vi "INTELLIFAUCET Driver.vi"(0 "VISA session":refnum<visa-resource-name>="MW100", 1 "Mode":T2=enum."Stop Flow", 2 "Use General Conversion":bool, 5 "Temperature(F)":dbl(slide)=58.0 scale=40.0..120.0, 7 "Flow Rate (GPM)":dbl(slide)=100.0 scale=0.0..100.0, 9 "uA Set":i32, 11 "Error In":errorcluster, 12 "Debug":bool, 13 "Refnum in":T1, 14 "Use Proportion Valve":bool) -> (4 "VISA session out":refnum<visa-resource-name>, 6 "Intellif Valve % Open":dbl, 8 "uA Output":i32, 15 "Error Out":errorcluster)   [LabVIEW 2016]
uses:
  Type Definitions/INTELLIFAUCET Set Mode.ctl
  Type Definitions/INTELLIFAUCT Temp Flow.ctl
panel:
  in  "milliseconds to wait":u32=25
  out "Local?":bool
  # "%"
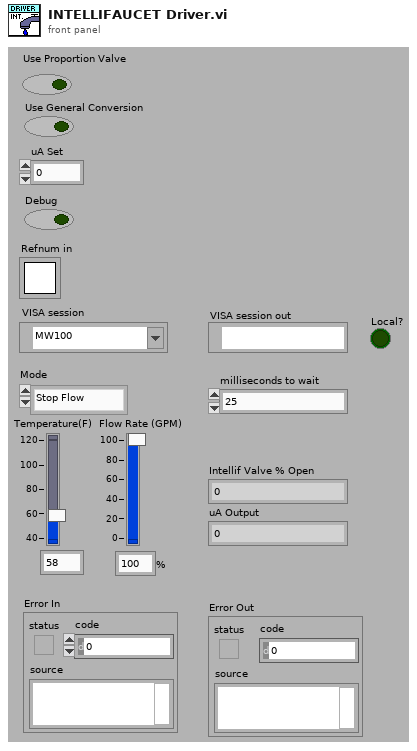
[diagram p1: front panel]
types:
  T1 = typedef "Semaphore RefNum" = refnum<k1>
  T2 = typedef "INTELLIFAUCET Set Mode.ctl" = enum16{"Adjust Temp", "Adjust Flow", "Start Flow", "Stop Flow", "Hold"}
  T3 = typedef "INTELLIFAUCT Temp Flow.ctl" = enum8{"TEMP", "FLOW"}
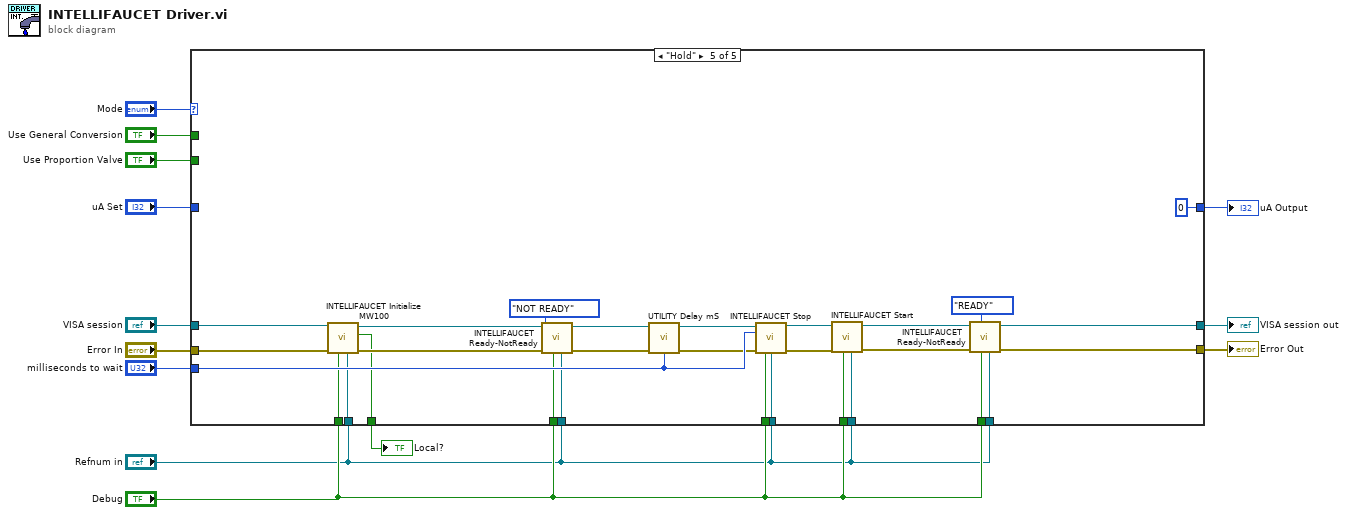
[diagram p0: block diagram]
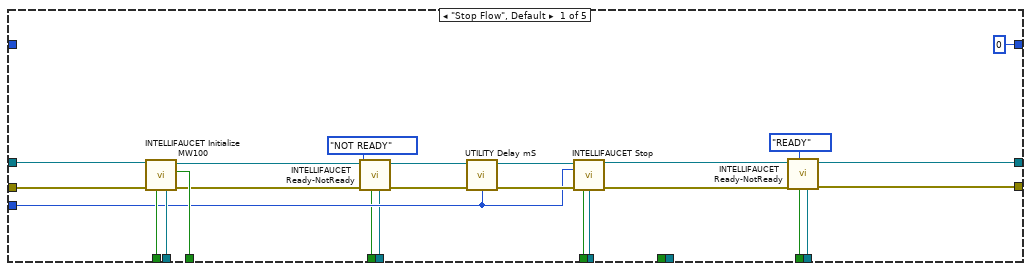
[diagram p2: hidden frame]
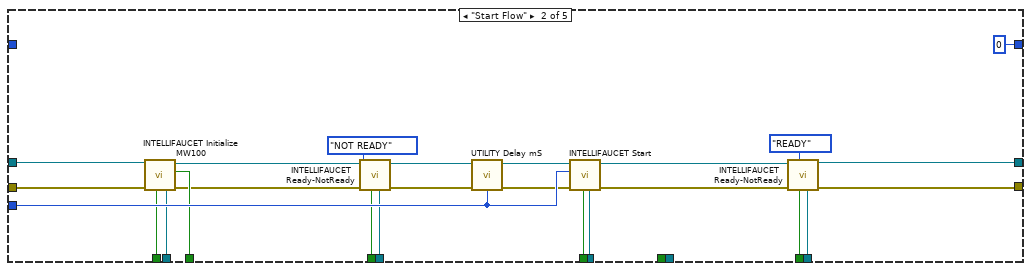
[diagram p3: hidden frame]
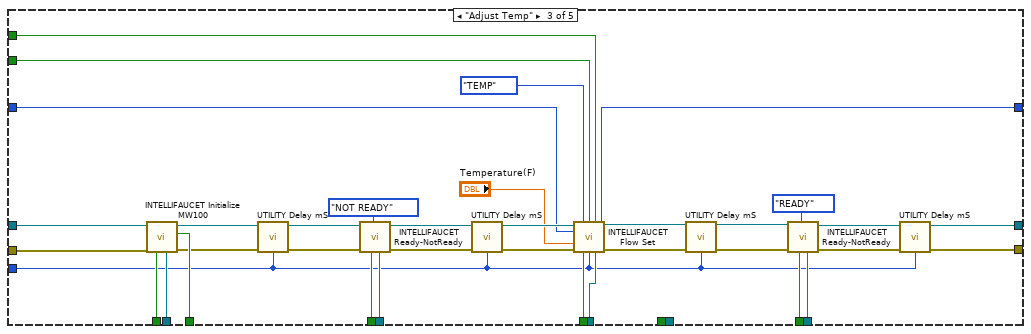
[diagram p4: hidden frame]
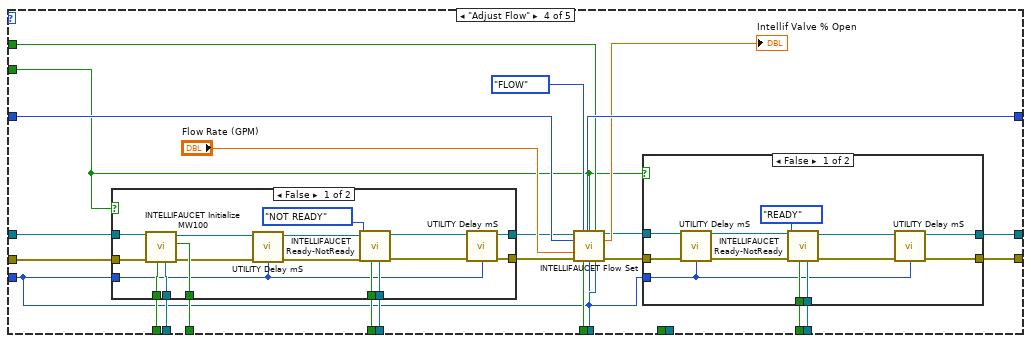
[diagram p5: hidden frame]
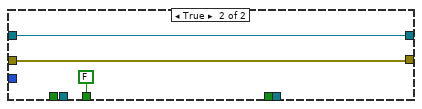
[diagram p7: hidden frame]
diagram:
  n1 = case shown="\"Hold\"" "Mode" {
    tunnel: "milliseconds to wait" -> [w28 w61 w65 w102 w168]
    tunnel: [w16 w46 w86 w115 w159] -> w10
    tunnel: "VISA session" -> [w35 w60 w84 w118 w170]
    tunnel: "Error In" -> [w36 w59 w85 w112 w169]
    tunnel: [w17 w45 w82 w117 w160] -> w11
    tunnel: [w34 w58 w81 w116 w163] -> w9
    tunnel: "Debug" -> [w26 w44 w78 w110 w165]
    tunnel: "Refnum in" -> [w25 w43 w77 w111 w164]
    tunnel: "Refnum in" -> [w32 w57 w79 w114 w166]
    tunnel: "Debug" -> [w33 w56 w80 w113 w167]
    tunnel: "Refnum in" -> [w30 w54 w75 w109 w161]
    tunnel: "Debug" -> [w31 w55 w76 w108 w162]
    tunnel: "Debug" -> [w15 w42 w74 w107 w158]
    tunnel: "Refnum in" -> [w14 w41 w73 w106 w157]
    tunnel: [0 ("uA Output") 0 ("uA Output") w72 w105 0 ("uA Output")] -> w8
    tunnel: "Use General Conversion" -> [_ _ w71 w103 _]
    tunnel: "uA Set" -> [_ _ w70 w104 _]
    tunnel: "Use Proportion Valve" -> [_ _ w62 w94 _]
    tunnel: "Debug" -> [_ _ _ _ w151]
    tunnel: "Refnum in" -> [_ _ _ _ w150]
    frame "Stop Flow", Default {
      n2 = call "INTELLIFAUCET Initialize MW100.vi"("Refnum in"=w32, "Debug"=w33, "error in (no error)"=w36, "MW100 Input"=w35) -> ("error out"=w24:errorcluster, "Local?"=w34:bool, "MW100 Output"=w22:refnum<visa-resource-name>)  [unwired: 5 in]
      n3 = call "INTELLIFAUCET Ready-NotReady.vi"("Refnum in"=w25, "Debug"=w26, "Error In"=w24, "READY?"=enum8{"READY", "NOT READY"}."NOT READY", "VISA session"=w22) -> ("Error Out"=w23:errorcluster, "dup VISA session"=w21:refnum<visa-resource-name>)  [unwired: 5 in]
      n4 = call "UTILITY Delay mS.vi"("Error In"=w23, "milliseconds to wait"=w28) -> ("Error Out"=w37:errorcluster)  [unwired: 13 in]
      n5 = call "INTELLIFAUCET Stop.vi"("VISA session"=w21, "mS wait"=w28, "Error In"=w37, "Debug"=w31, "Refnum in"=w30) -> ("dup VISA session"=w19:refnum<visa-resource-name>, "Error Out"=w18:errorcluster)  [unwired: 9 in]
      n6 = call "INTELLIFAUCET Ready-NotReady.vi"("Refnum in"=w14, "Debug"=w15, "Error In"=w18, "READY?"=enum8{"READY", "NOT READY"}."READY", "VISA session"=w19) -> ("Error Out"=w16:errorcluster, "dup VISA session"=w17:refnum<visa-resource-name>)  [unwired: 5 in]
    }
    frame "Start Flow" {
      n7 = call "INTELLIFAUCET Initialize MW100.vi"("Refnum in"=w57, "Debug"=w56, "error in (no error)"=w59, "MW100 Input"=w60) -> ("error out"=w38:errorcluster, "Local?"=w58:bool, "MW100 Output"=w51:refnum<visa-resource-name>)  [unwired: 5 in]
      n8 = call "INTELLIFAUCET Ready-NotReady.vi"("Refnum in"=w43, "Debug"=w44, "Error In"=w38, "READY?"=enum8{"READY", "NOT READY"}."NOT READY", "VISA session"=w51) -> ("Error Out"=w40:errorcluster, "dup VISA session"=w50:refnum<visa-resource-name>)  [unwired: 5 in]
      n9 = call "UTILITY Delay mS.vi"("Error In"=w40, "milliseconds to wait"=w61) -> ("Error Out"=w39:errorcluster)  [unwired: 13 in]
      n10 = call "INTELLIFAUCET Start.vi"("Refnum in"=w54, "Debug"=w55, "Error In"=w39, "mS wait"=w61, "VISA session"=w50) -> ("Error Out"=w47:errorcluster, "dup VISA session"=w48:refnum<visa-resource-name>)  [unwired: 5 in]
      n11 = call "INTELLIFAUCET Ready-NotReady.vi"("Refnum in"=w41, "Debug"=w42, "Error In"=w47, "READY?"=enum8{"READY", "NOT READY"}."READY", "VISA session"=w48) -> ("Error Out"=w46:errorcluster, "dup VISA session"=w45:refnum<visa-resource-name>)  [unwired: 5 in]
    }
    frame "Adjust Temp" {
      n12 = call "INTELLIFAUCET Initialize MW100.vi"("Refnum in"=w79, "Debug"=w80, "error in (no error)"=w85, "MW100 Input"=w84) -> ("error out"=w67:errorcluster, "Local?"=w81:bool, "MW100 Output"=w83:refnum<visa-resource-name>)  [unwired: 5 in]
      n13 = call "UTILITY Delay mS.vi"("Error In"=w67, "milliseconds to wait"=w65) -> ("Error Out"=w66:errorcluster)  [unwired: 13 in]
      n14 = call "INTELLIFAUCET Ready-NotReady.vi"("Refnum in"=w77, "Debug"=w78, "Error In"=w66, "READY?"=enum8{"READY", "NOT READY"}."NOT READY", "VISA session"=w83) -> ("Error Out"=w69:errorcluster, "dup VISA session"=w91:refnum<visa-resource-name>)  [unwired: 5 in]
      n15 = call "UTILITY Delay mS.vi"("Error In"=w69, "milliseconds to wait"=w65) -> ("Error Out"=w68:errorcluster)  [unwired: 13 in]
      n16 = call "INTELLIFAUCET Flow Set.vi"("VISA Refnum in"=w91, "TEMP,FLOW"=INTELLIFAUCT_Temp_Flow."TEMP", "Use Proportion Valve"=w62, "Use General Conversion"=w71, "uA Set"=w70, "Temp/GPM Target"="Temperature(F)", "error in (no error)"=w68, "Debug"=w76, "milliseconds to wait"=w65, "Refnum in"=w75) -> ("VISA Refnum out"=w88:refnum<visa-resource-name>, "uA Output"=w72:i32, "error out"=w92:errorcluster)  [unwired: 2 in, 1 out]
      n17 = call "UTILITY Delay mS.vi"("Error In"=w92, "milliseconds to wait"=w65) -> ("Error Out"=w87:errorcluster)  [unwired: 13 in]
      n18 = call "INTELLIFAUCET Ready-NotReady.vi"("Refnum in"=w73, "Debug"=w74, "Error In"=w87, "READY?"=enum8{"READY", "NOT READY"}."READY", "VISA session"=w88) -> ("Error Out"=w89:errorcluster, "dup VISA session"=w82:refnum<visa-resource-name>)  [unwired: 5 in]
      n19 = call "UTILITY Delay mS.vi"("Error In"=w89, "milliseconds to wait"=w65) -> ("Error Out"=w86:errorcluster)  [unwired: 13 in]
    }
    frame "Adjust Flow" {
      n20 = case shown="False" w94 {
        tunnel: w118 -> [w145 w147]
        tunnel: [w144 FALSE ("Local?")] -> w116
        tunnel: w114 -> [w143 _]
        tunnel: w113 -> [w142 _]
        tunnel: w112 -> [w141 w148]
        tunnel: w111 -> [w140 _]
        tunnel: w110 -> [w139 _]
        tunnel: w102 -> [w138 _]
        tunnel: [w136 w147] -> w98
        tunnel: [w134 w148] -> w95
        frame False {
          n21 = call "INTELLIFAUCET Initialize MW100.vi"("Refnum in"=w143, "Debug"=w142, "error in (no error)"=w141, "MW100 Input"=w145) -> ("error out"=w133:errorcluster, "Local?"=w144:bool, "MW100 Output"=w137:refnum<visa-resource-name>)  [unwired: 5 in]
          n22 = call "UTILITY Delay mS.vi"("Error In"=w133, "milliseconds to wait"=w138) -> ("Error Out"=w132:errorcluster)  [unwired: 13 in]
          n23 = call "INTELLIFAUCET Ready-NotReady.vi"("Refnum in"=w140, "Debug"=w139, "Error In"=w132, "READY?"=enum8{"READY", "NOT READY"}."NOT READY", "VISA session"=w137) -> ("Error Out"=w135:errorcluster, "dup VISA session"=w136:refnum<visa-resource-name>)  [unwired: 5 in]
          n24 = call "UTILITY Delay mS.vi"("Error In"=w135, "milliseconds to wait"=w138) -> ("Error Out"=w134:errorcluster)  [unwired: 13 in]
        }
        frame True {
        }
      }
      n25 = call "INTELLIFAUCET Flow Set.vi"("VISA Refnum in"=w98, "TEMP,FLOW"=INTELLIFAUCT_Temp_Flow."FLOW", "Use Proportion Valve"=w94, "Use General Conversion"=w103, "uA Set"=w104, "Temp/GPM Target"="Flow Rate (GPM)", "error in (no error)"=w95, "Debug"=w108, "milliseconds to wait"=w102, "Refnum in"=w109) -> ("VISA Refnum out"=w97:refnum<visa-resource-name>, "Valve % Open"=→"Intellif Valve % Open":dbl, "uA Output"=w105:i32, "error out"=w96:errorcluster)  [unwired: 2 in]
      n26 = case shown="False" w94 {
        tunnel: [w128 w130] -> w117
        tunnel: [w127 w129] -> w115
        tunnel: w107 -> [w126 _]
        tunnel: w106 -> [w125 _]
        tunnel: w102 -> [w124 _]
        tunnel: w97 -> [w121 w130]
        tunnel: w96 -> [w120 w129]
        frame False {
          n27 = call "UTILITY Delay mS.vi"("Error In"=w120, "milliseconds to wait"=w124) -> ("Error Out"=w122:errorcluster)  [unwired: 13 in]
          n28 = call "INTELLIFAUCET Ready-NotReady.vi"("Refnum in"=w125, "Debug"=w126, "Error In"=w122, "READY?"=enum8{"READY", "NOT READY"}."READY", "VISA session"=w121) -> ("Error Out"=w123:errorcluster, "dup VISA session"=w128:refnum<visa-resource-name>)  [unwired: 5 in]
          n29 = call "UTILITY Delay mS.vi"("Error In"=w123, "milliseconds to wait"=w124) -> ("Error Out"=w127:errorcluster)  [unwired: 13 in]
        }
        frame True {
        }
      }
    }
    frame "Hold" {
      n30 = call "INTELLIFAUCET Initialize MW100.vi"("Refnum in"=w166, "Debug"=w167, "error in (no error)"=w169, "MW100 Input"=w170) -> ("error out"=w175:errorcluster, "Local?"=w163:bool, "MW100 Output"=w173:refnum<visa-resource-name>)  [unwired: 5 in]
      n31 = call "INTELLIFAUCET Ready-NotReady.vi"("Refnum in"=w164, "Debug"=w165, "Error In"=w175, "READY?"=enum8{"READY", "NOT READY"}."NOT READY", "VISA session"=w173) -> ("Error Out"=w174:errorcluster, "dup VISA session"=w172:refnum<visa-resource-name>)  [unwired: 5 in]
      n32 = call "UTILITY Delay mS.vi"("Error In"=w174, "milliseconds to wait"=w168) -> ("Error Out"=w152:errorcluster)  [unwired: 13 in]
      n33 = call "INTELLIFAUCET Stop.vi"("VISA session"=w172, "mS wait"=w168, "Error In"=w152, "Debug"=w162, "Refnum in"=w161) -> ("dup VISA session"=w156:refnum<visa-resource-name>, "Error Out"=w154:errorcluster)  [unwired: 9 in]
      n34 = call "INTELLIFAUCET Start.vi"("Refnum in"=w150, "Debug"=w151, "Error In"=w154, "VISA session"=w156) -> ("Error Out"=w153:errorcluster, "dup VISA session"=w155:refnum<visa-resource-name>)  [unwired: 6 in]
      n35 = call "INTELLIFAUCET Ready-NotReady.vi"("Refnum in"=w157, "Debug"=w158, "Error In"=w153, "READY?"=enum8{"READY", "NOT READY"}."READY", "VISA session"=w155) -> ("Error Out"=w159:errorcluster, "dup VISA session"=w160:refnum<visa-resource-name>)  [unwired: 5 in]
    }
  }
  "Error Out" <- w10
  "VISA session out" <- w11
  "Local?" <- w9
  "uA Output" <- w8
